vi "Set Error State.vi"(8 "error in (no error)":errorcluster, 11 "Process in":refnum<class "Process.lvclass">) -> (0 "error out":errorcluster, 3 "Process out":refnum<class "Process.lvclass">)   [LabVIEW 2019, in "TelemetryAsync Engine.lvlib" / "Process.lvclass"]
uses:
  Process.lvclass
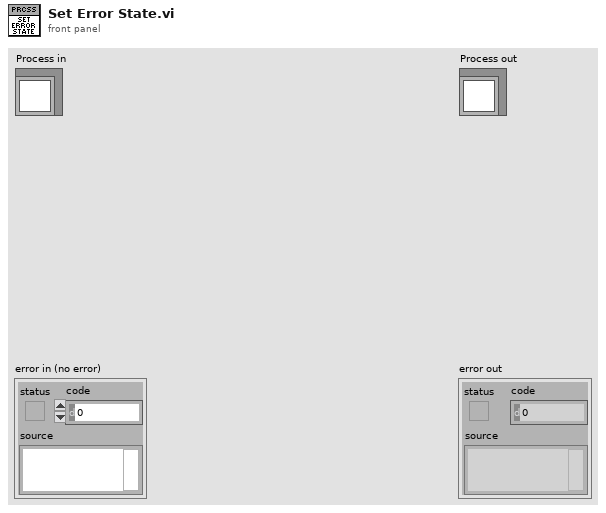
[diagram p1: front panel]
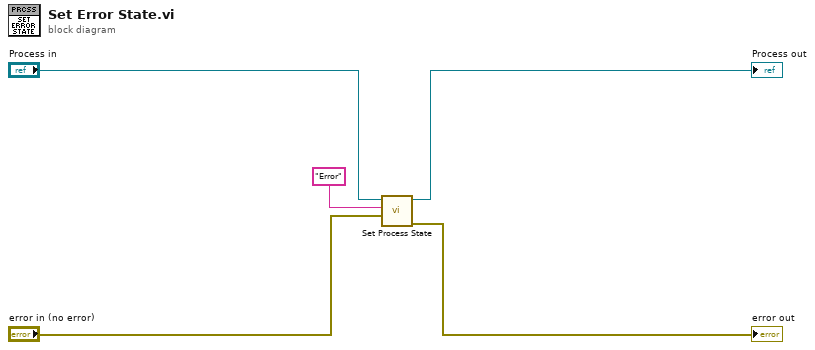
[diagram p0: block diagram]
diagram:
  n1 = call "Set Process State.vi"("Payload"="error in (no error)", "Command"="Error", "Process in"="Process in") -> ("error out"=→"error out":errorcluster, "Process out"=→"Process out":refnum<class "Process.lvclass">)  [unwired: 7 in]
